vi "Open Item Reference.vi"(8 "error in (no error)":errorcluster, 10 "App Ref (local)":refnum<vi>, 11 "VI in":refnum<class "VI.lvclass">) -> (0 "error out":errorcluster, 3 "VI out":refnum<class "VI.lvclass">)   [LabVIEW 2020, in "VI Properties Editor.lvlib" / "VI.lvclass"]
doc: "Opens a reference to <B>VI in</B>."
uses:
  VI.lvclass
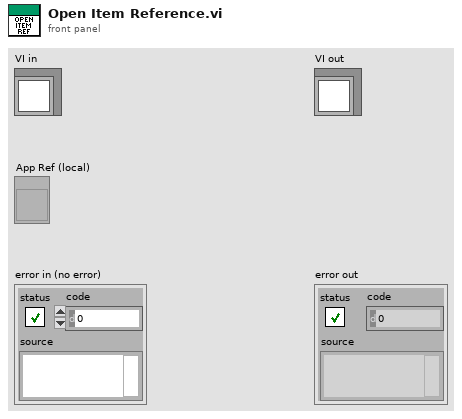
[diagram p1: front panel]
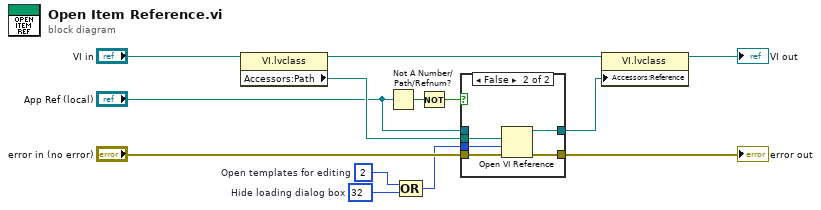
[diagram p0: block diagram]
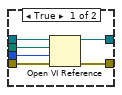
[diagram p2: hidden frame]
diagram:
  w5 = 32  # Hide loading dialog box
  w6 = 2  # Open templates for editing
  n1 = property class="VI.lvclass"(reference="VI in") -> (reference out=w12:refnum<class "VI.lvclass">, "Accessors:Path"=w10:path)  [unwired: 1 in, 1 out]
  n2 = Not A Number/Path/Refnum?(number/path/refnum="App Ref (local)") -> (NaN/Path/Refnum?=w2:bool)
  n3 = Compound Arithmetic op=OR(w6, w5) -> (w4:i32)
  n4 = Not(x=w2) -> (.not. x?=w1:bool)
  n5 = case shown="False" w1 {
    tunnel: w10 -> [w19 w24]
    tunnel: "error in (no error)" -> [w18 w23]
    tunnel: [w17 w22] -> w8
    tunnel: [w16 w21] -> w7
    tunnel: w4 -> [w15 w20]
    tunnel: "App Ref (local)" -> [w14 _]
    frame True {
      n6 = Open VI Reference(application reference (local)=w14, vi path=w19, options=w15, error in (no error)=w18) -> (vi reference=w16:refnum<vi>, error out=w17:errorcluster)  [unwired: 2 in]
    }
    frame False {
      n7 = Open VI Reference(vi path=w24, options=w20, error in (no error)=w23) -> (vi reference=w21:refnum<vi>, error out=w22:errorcluster)  [unwired: 3 in]
    }
  }
  "error out" <- w8
  n8 = property class="VI.lvclass"(reference=w12, "Accessors:Reference"=w7) -> (reference out=→"VI out":refnum<class "VI.lvclass">)  [unwired: 1 in, 1 out]
